vi "CAN Read Setting.vi"(8 "error in (no error)":errorcluster, 11 "Instrument Parameter":string[][](array[string])) -> (0 "error out":errorcluster, 2 "CAN Output":T1 {"data"."payload" format="%x"; "data"."timestamp" format="%<%.7X\n%x>T"; "data"."type" items=["CAN Data"=0, "CAN Remote"=1, "CAN Bus Error"=2, "CAN 2.0 Data"=8, "CAN FD Data"=16, "CAN FD+BRS Data"=24, "J1939 Data"=192, "Delay"=224, "Log Trigger"=225, "Start Trigger"=226]; "data"."identifier" format="%x"}, 3 "CAN Input":T4)   [LabVIEW 2021, in "CAN.lvlib"]
uses:
  CAN.lvlib
  CAN Input.ctl
  CAN Output.ctl
  <vilib>/xnet/xnet.llb/XNET Frame CAN.ctl
  <vilib>/xnet/xnet.llb/XNET Frame Type CAN.ctl
  User Interface/User Interface.lvlib
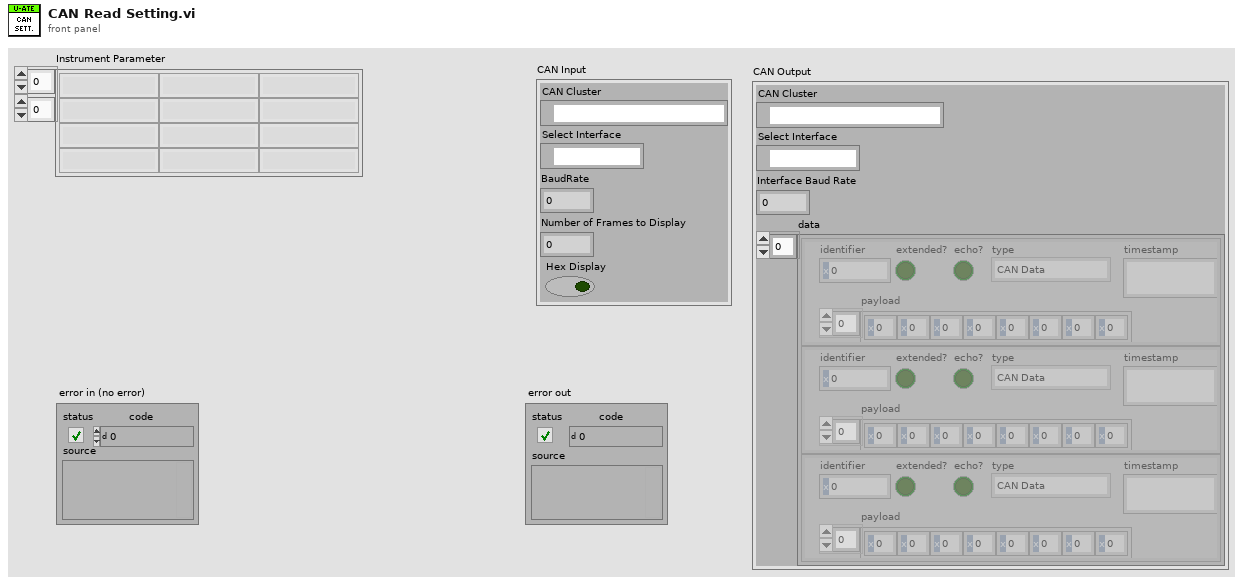
[diagram p1: front panel]
types:
  T1 = typedef "CAN.lvlib/CAN Output.ctl" = cluster{"CAN Cluster":refnum<k21>, "Select Interface":refnum<k21>, "Interface Baud Rate":u32, "data":T2[]}
  T2 = typedef "XNET Frame CAN.ctl" = cluster{"timestamp":timestamp, "payload":u8[], "identifier":u32, "type":T3, "extended?":bool, "echo?":bool}
  T3 = typedef "XNET Frame Type CAN.ctl" = u8
  T4 = typedef "CAN.lvlib/CAN Input.ctl" = cluster{"CAN Cluster":refnum<k21>, "Select Interface":refnum<k21>, "BaudRate":u32, "Number of Frames to Display":i32, "Hex Display":bool}
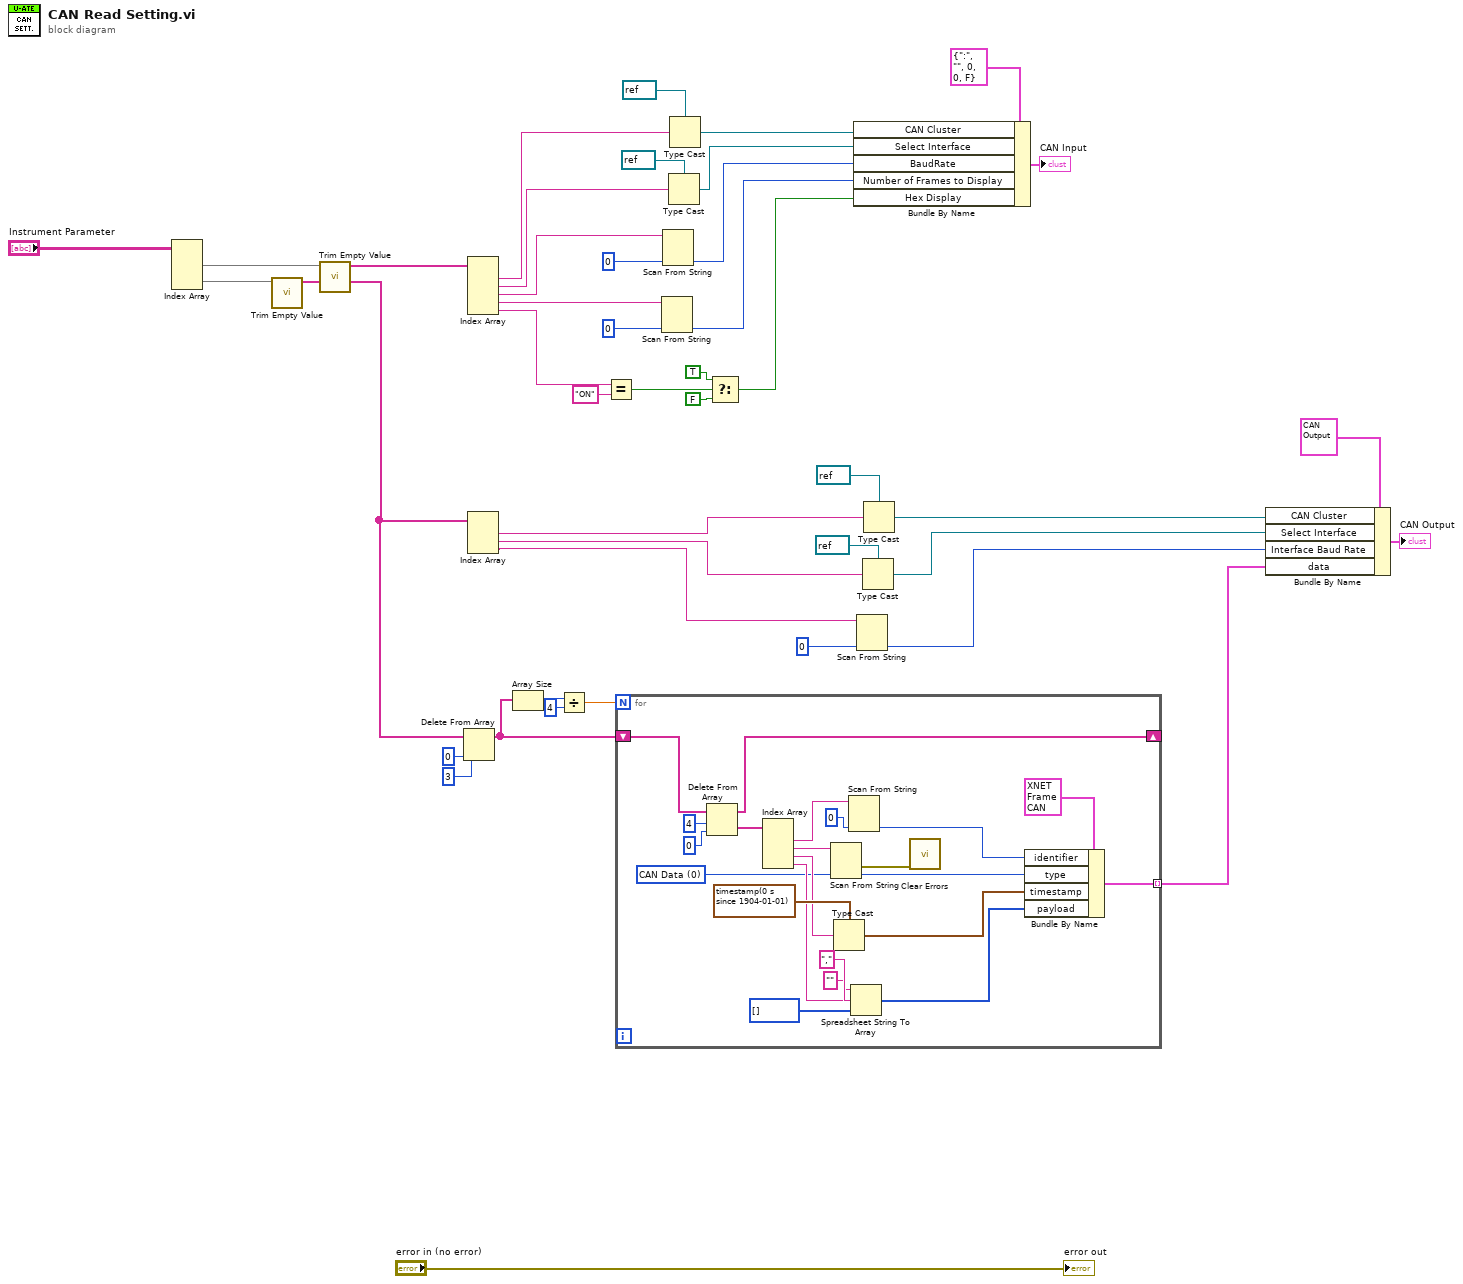
[diagram p0: block diagram]
diagram:
  n1 = Index Array(array="Instrument Parameter") -> (element #1=w42:string[], element #2=w41:string[])  [unwired: 4 in]
  n2 = call "Trim Empty Value.vi"("Data In"=w41) -> ("Data Out"=w15:string[])  [unwired: 10 in]
  n3 = call "Trim Empty Value.vi"("Data In"=w42) -> ("Data Out"=w14:string[])  [unwired: 10 in]
  n4 = Delete From Array(array=w15, length=3, index=0) -> (array with subset deleted=w19:string[])  [unwired: 1 out]
  n5 = Index Array(array=w14) -> (element #1=w40:string, element #2=w39:string, element #3=w31:string, element #4=w29:string, element #5=w37:string)  [unwired: 5 in]
  n6 = Index Array(array=w15) -> (element #1=w24:string, element #2=w23:string, element #3=w22:string)  [unwired: 3 in]
  n7 = Array Size(array=w19) -> (size(s)=w18:i32)
  n8 = Divide(x=w18, y=4) -> (x/y=w16:dbl)
  n9 = Equal?(x=w37, y="ON") -> (x = y?=w35:bool)
  n10 = for {
    N: w16 -> [_]
    shift-right: [w63] -> _
    shift-left: w19 -> [w66]
    tunnel: [w48] -> w2 mode=indexing
    w46 = T3 0 items=["CAN Data"=0, "CAN Remote"=1, "CAN Bus Error"=2, "CAN 2.0 Data"=8, "CAN FD Data"=16, "CAN FD+BRS Data"=24, "J1939 Data"=192, "Delay"=224, "Log Trigger"=225, "Start Trigger"=226] ("CAN frame.type")
    n11 = Delete From Array(array=w66, length=4, index=0) -> (deleted portion=w62:string[], array with subset deleted=w63:string[])
    n12 = Index Array(array=w62) -> (element #1=w61:string, element #2=w58:string, element #3=w55:string, element #4=w50:string)  [unwired: 4 in]
    n13 = Scan From String(input string=w58, default 1=w46) -> (error out=w47:errorcluster, output 1=w57:T3)  [unwired: 3 in, 2 out]
    n14 = Type Cast(type=timestamp(0 s since 1904-01-01) ("CAN frame.timestamp"), x=w55) -> (*(type *) &x=w54:timestamp)
    n15 = Scan From String(input string=w61, default 1=u32 0 ("CAN frame.identifier")) -> (output 1=w59:u32)  [unwired: 3 in, 3 out]
    n16 = Spreadsheet String To Array(delimiter (Tab)=",", format string="", spreadsheet string=w50, array type (2D Dbl)=u8[] [] ("CAN frame.payload")) -> (array=w49:u8[])
    n17 = call <vilib>:"Clear Errors.vi"("error in (no error)"=w47) -> ()  [unwired: 5 in, 2 out]
    n18 = Bundle By Name(cluster=T2 {"timestamp"=timestamp(0 s since 1904-01-01), "payload"=[], "identifier"=0, "type"=0, "extended?"=FALSE, "echo?"=FALSE} ("CAN frame"), "identifier"=w59, "type"=w57, "timestamp"=w54, "payload"=w49) -> (w48:T2)
  }
  n19 = Scan From String(input string=w29, default 1=0 ("Number of Frames to Display")) -> (output 1=w9:i32)  [unwired: 3 in, 3 out]
  n20 = Scan From String(input string=w31, default 1=u32 0 ("BaudRate")) -> (output 1=w10:u32)  [unwired: 3 in, 3 out]
  n21 = Type Cast(type=refnum<k21> refnum ("Select Interface"), x=w39) -> (*(type *) &x=w11:refnum<k21>)
  n22 = Type Cast(type=refnum<k21> refnum ("CAN Cluster"), x=w40) -> (*(type *) &x=w12:refnum<k21>)
  n23 = Select(t=TRUE, s=w35, f=FALSE) -> (s? t:f=w8:bool)
  n24 = Bundle By Name(cluster=T4 {"CAN Cluster"=":", "Select Interface"="", "BaudRate"=0, "Number of Frames to Display"=0, "Hex Display"=FALSE} ("CAN Input"), "CAN Cluster"=w12, "Select Interface"=w11, "BaudRate"=w10, "Number of Frames to Display"=w9, "Hex Display"=w8) -> (→"CAN Input":T4)
  n25 = Scan From String(input string=w22, default 1=u32 0 ("BaudRate")) -> (output 1=w3:u32)  [unwired: 3 in, 3 out]
  n26 = Type Cast(type=refnum<k21> refnum ("Select Interface"), x=w23) -> (*(type *) &x=w4:refnum<k21>)
  n27 = Type Cast(type=refnum<k21> refnum ("CAN Cluster"), x=w24) -> (*(type *) &x=w5:refnum<k21>)
  n28 = Bundle By Name(cluster=T1 {"CAN Cluster"=":memory:", "Select Interface"="CAN1", "Interface Baud Rate"=125000, "data"=[{"timestamp"=timestamp(0 s since 1904-01-01), "payload"=[1, 2, 3, 4, 5, 6, 7, 8], "identifier"=2, "type"=0, "extended?"=FALSE, "echo?"=FALSE}, {"timestamp"=timestamp(0 s since 1904-01-01), "payload"=[0, 1, 2, 3, 4, 5, 6, 7], "identifier"=3, "type"=0, "extended?"=FALSE, "echo?"=FALSE}]} ("CAN Output"), "CAN Cluster"=w5, "Select Interface"=w4, "Interface Baud Rate"=w3, "data"=w2) -> (→"CAN Output":T1)
  "error out" <- "error in (no error)"
